vi "McPherson display color.vi"(0 "Current":dbl format="%.5f", 1 "Start":dbl format="%.2f", 2 "End":dbl format="%.2f") -> (3 "Current":cluster{dbl, dbl}(slide)={0.0, -0.0065359477124182705} scale=695.0..764.5 scale format="%.1f", 4 "Fill Color":u32 format="%.0x", 5 "PercentDone":sgl min=0 max=100 format="%.1f", 6 "Fill Style":u32)   [LabVIEW 2020]
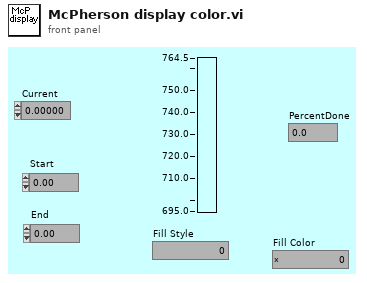
[diagram p1: front panel]
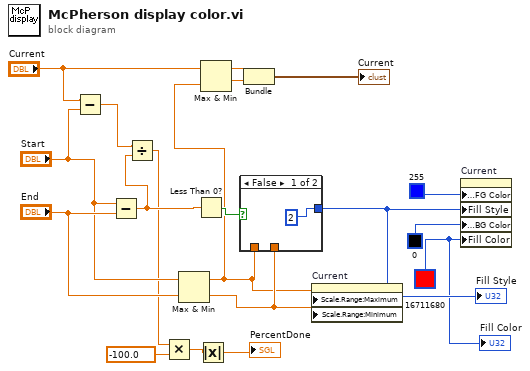
[diagram p0: block diagram]
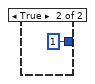
[diagram p2: hidden frame]
diagram:
  w1 = u32 16711680
  n1 = Subtract(x="Current", y="Start") -> (x-y=w7:dbl)
  n2 = Subtract(x="Start", y="End") -> (x-y=w6:dbl)
  n3 = Divide(x=w7, y=w6) -> (x/y=w5:dbl)
  n4 = Multiply(x=w5, y=-100.0) -> (x*y=w3:dbl)
  n5 = Max & Min(x="Start", y="End") -> (max(x,y)=w12:dbl, min(x,y)=w14:dbl)
  n6 = Less Than 0?(x=w6) -> (x < 0?=w15:bool)
  n7 = Absolute Value(x=w3) -> (abs(x)=→"PercentDone":dbl)
  n8 = Max & Min(x="Current", y=w12) -> (max(x,y)=w18:dbl, min(x,y)=w17:dbl)
  n9 = case shown="False" w15 {
    tunnel: w12 -> [_ _]
    tunnel: w14 -> [_ _]
    tunnel: [2 ("Write Attribute") 1 ("Write Attribute")] -> w10
    frame False {
    }
    frame True {
    }
  }
  "Fill Style" <- w10
  n10 = Bundle(w18, w17) -> (→"Current":cluster{dbl, dbl})  [unwired: 1 in]
  n11 = property on="Current" class="Slide (strict)"("Scale.Range:Maximum"=w12, "Scale.Range:Minimum"=w14) -> ()  [unwired: 2 in, 2 out]
  n12 = property on="Current" class="Slide (strict)"("Slider Colors:FG Color"=u32 255, "Fill Style"=w10, "Slider Colors:BG Color"=u32 0, "Fill Color"=w1) -> ()  [unwired: 2 in, 2 out]
  "Fill Color" <- w1
